vi "save_as.vi"(7 "calibration info":T1, 8 "Array":u16[][](array[numeric]), 9 "Camera":T2, 10 "Control Camera Properties 3":T3={"Packet Size"=1500, "Pixel Format"=17825797, "Gain in dB"=1.0, "Exposure Time in µs"=1500, "Stream Bytes per Second"=50000017} caption="Control Camera Properties" {"Stream Bytes per Second" min=1000000 max=124000000 step=100000 format="%.1p"; "Exposure Time in µs" min=21 max=153391689 format="%#.0f"; "Gain in dB" min=0.0 max=26.0 format="%#_2g"; "Pixel Format" items=["Mono 12 Packed"=17563654, "Mono 12"=17825797]}, 11 "path":path) -> (0 "saving error out":errorcluster, 2 "Name Time Date Out":string, 3 "Path out":path)   [LabVIEW 2014]
uses:
  type definitions/control camera properties.ctl
  type definitions/state machine enum.ctl
panel:
  out "Complete File Name Out":string
  in  "Time":bool
  in  "Date":bool
  in  "Name Time Date":string="im_spec" caption="Insert File Name"
  in  "Cancel Button":bool
  in  "Okay":bool
  in  "Path":path=path "C:/Users/loa/Documents/imaging-spectrometer/imaging-spectrometer/data"
  # "Tick box(es) to append time and/or date to file name:"
  # "Bytes"
  # "Trigger"
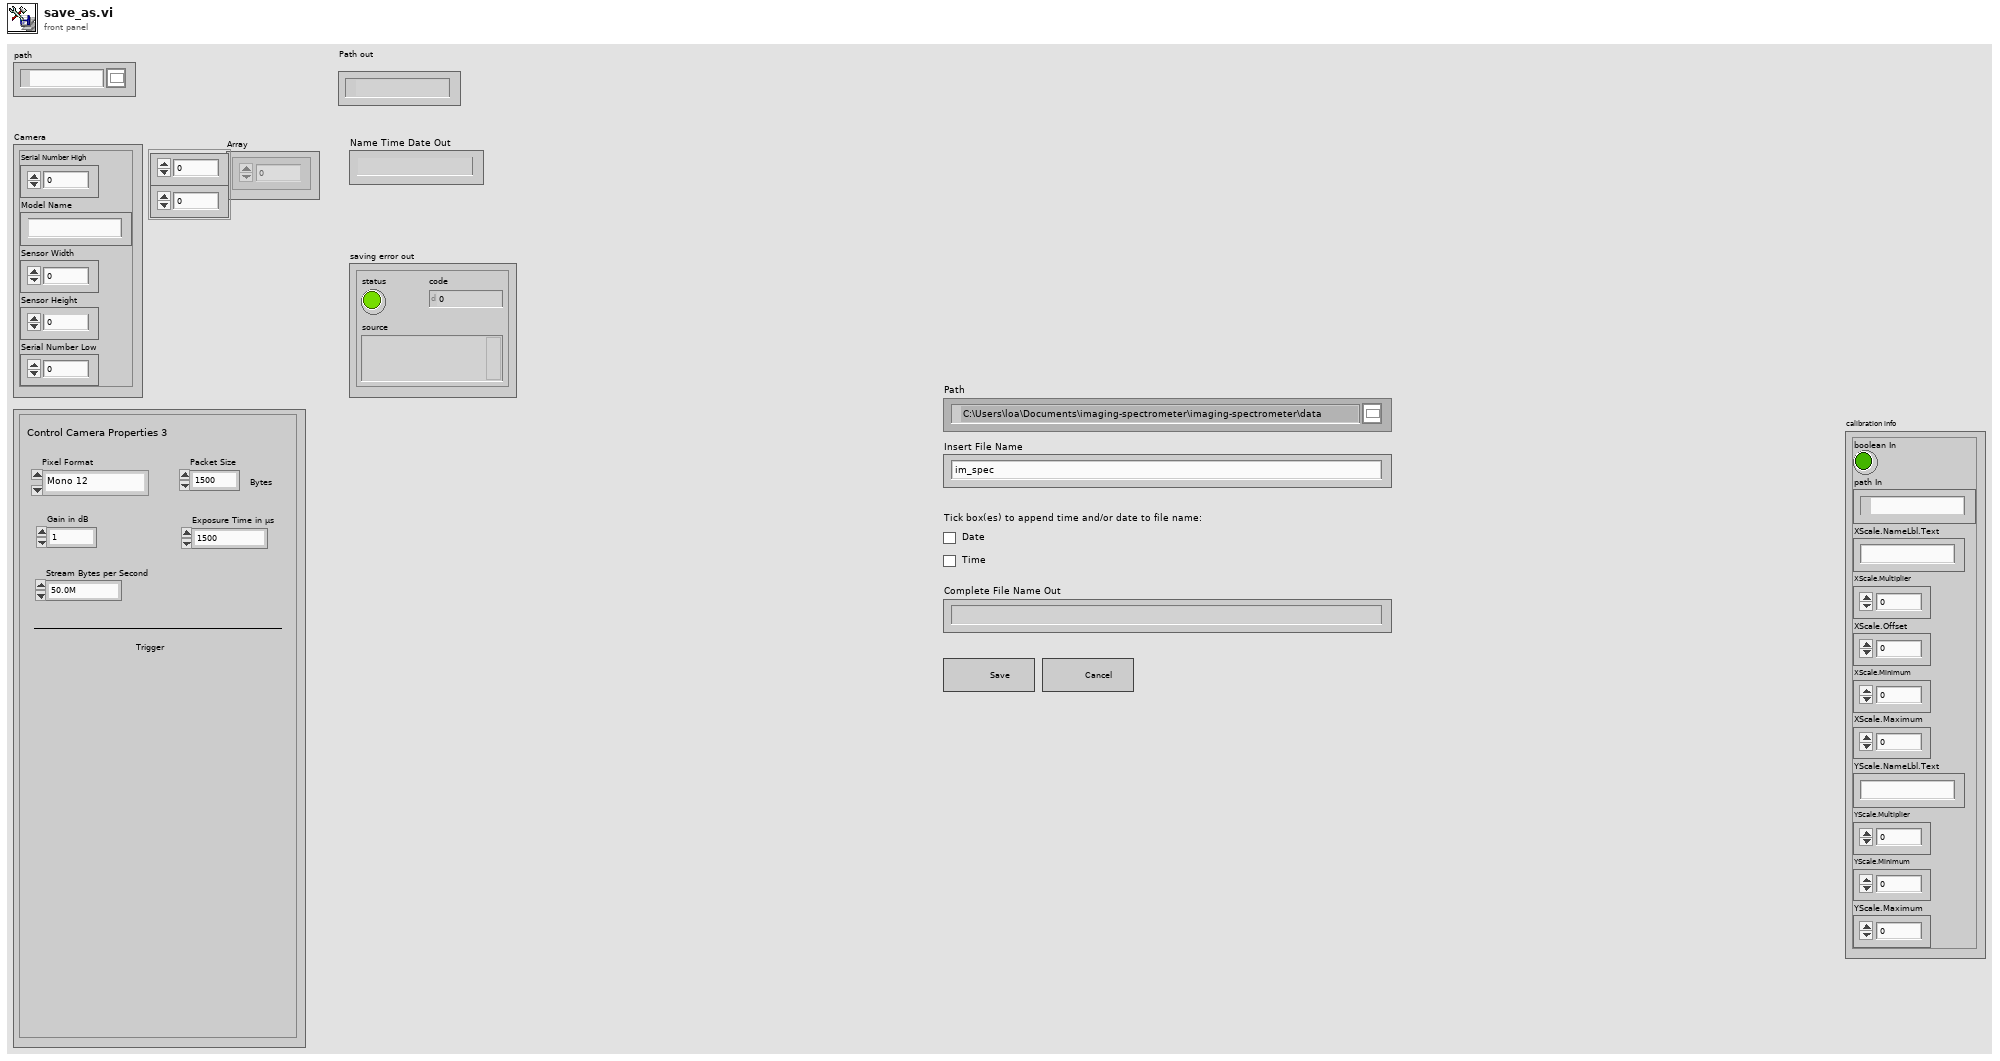
[diagram p1: front panel]
types:
  T1 = cluster{"boolean In":bool, "path In":path, "XScale.NameLbl.Text":string, "XScale.Multiplier":dbl, "XScale.Offset":dbl, "XScale.Minimum":dbl, "XScale.Maximum":dbl, "YScale.NameLbl.Text":string, "YScale.Multiplier":dbl, "YScale.Minimum":dbl, "YScale.Maximum":dbl}
  T2 = cluster{"Serial Number High":u32, "Model Name":string, "Sensor Width":u32, "Sensor Height":u32, "Serial Number Low":u32}
  T3 = typedef "control camera properties.ctl" = cluster{"Packet Size":u32, "Pixel Format":u32, "Gain in dB":dbl, "Exposure Time in µs":u32, "Stream Bytes per Second":u32}
  T4 = typedef "state machine enum.ctl" = enum16{"start", "select camera", "control camera properties", "calibration", "wait", "snap", "save", "save as", "grab", "error", "stop"}
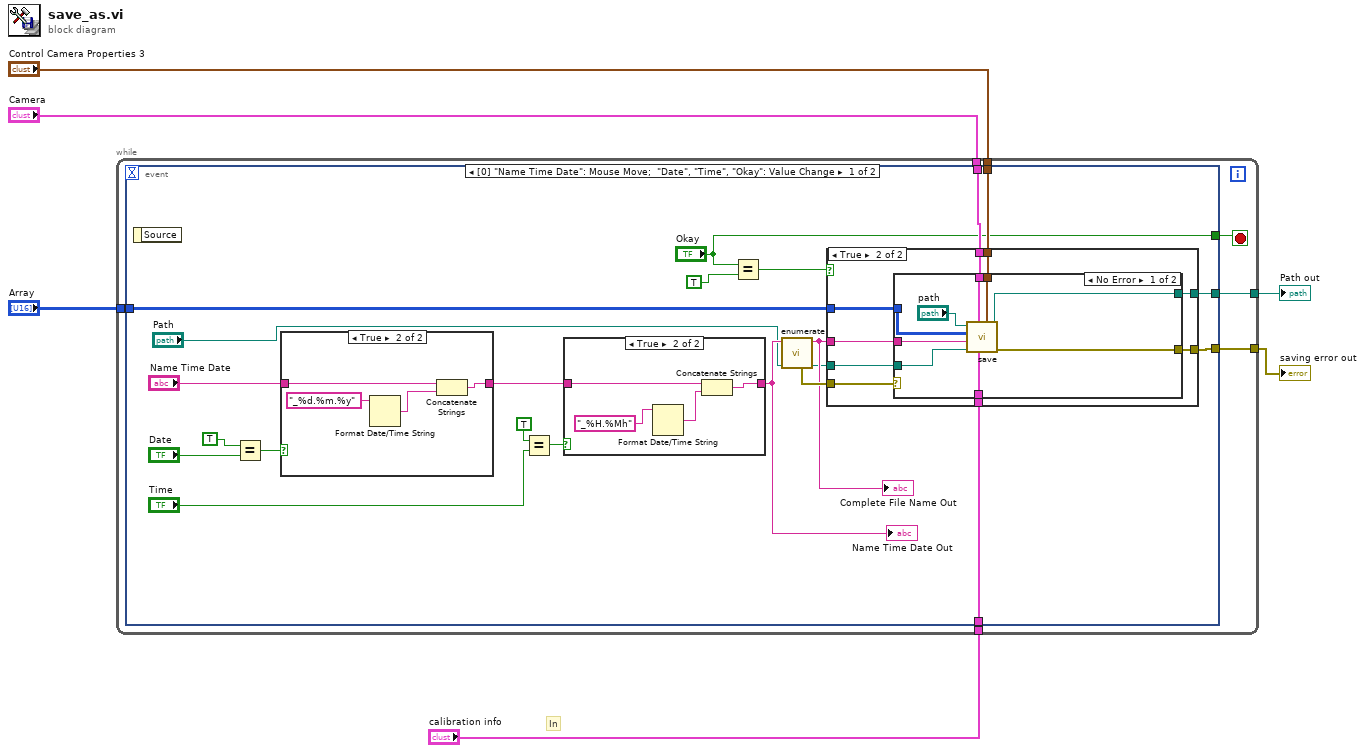
[diagram p0: block diagram]
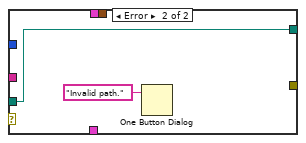
[diagram p3: hidden frame]
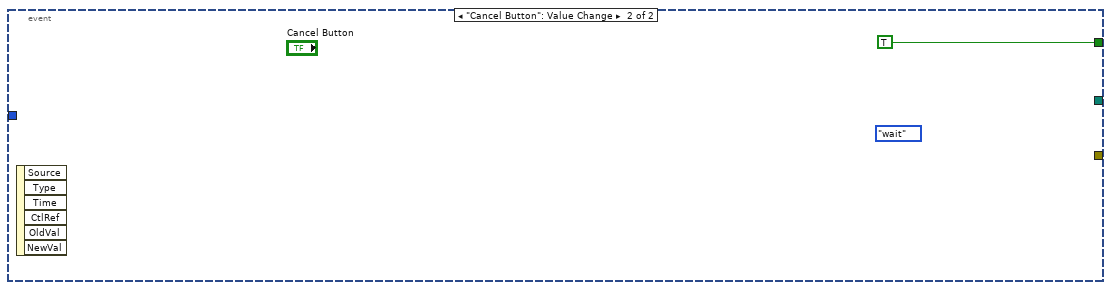
[diagram p6: hidden frame]
diagram:
  # "In"
  n1 = while {
    tunnel: "Control Camera Properties 3" -> [w12]
    tunnel: "Camera" -> [w11]
    tunnel: "Array" -> [w10]
    tunnel: [w9] -> w3
    tunnel: [w8] -> w2
    tunnel: "calibration info" -> [w7]
    stop <- w13 stop-if-true
    n2 = event shown="[0] \"Name Time Date\": Mouse Move;  \"Date\", \"Time\", \"Okay\": Value Change" {
      selector: _ -> [_ _]
      dyn-events: _ -> [_ _]
      timeout: _ -> [_ _]
      tunnel: ["Okay" TRUE] -> w13
      tunnel: w12 -> [w35 _]
      tunnel: w11 -> [w34 _]
      tunnel: w10 -> [w33 _]
      tunnel: [w32 _] -> w9
      tunnel: [w15 _] -> w8
      tunnel: w7 -> [w14 _]
      event "Name Time Date": Mouse Move; "Date", "Time", "Okay": Value Change {
        n3 = event-data() -> ()  [unwired: 1 in, 1 out]
        n4 = Equal?(x=TRUE, y="Date") -> (x = y?=w26:bool)
        n5 = case shown="True" w26 {
          tunnel: [w61 w64] -> w29
          tunnel: "Name Time Date" -> [w61 w62]
          frame False {
          }
          frame True {
            n6 = Format Date/Time String(time format string (%c)="_%d.%m.%y") -> (date/time string=w63:string)  [unwired: 2 in]
            n7 = Concatenate Strings(w62, w63) -> (w64:string)
          }
        }
        n8 = Equal?(x=TRUE, y="Time") -> (x = y?=w28:bool)
        n9 = case shown="True" w28 {
          tunnel: w29 -> [w56 w59]
          tunnel: [w56 w57] -> w21
          frame False {
          }
          frame True {
            n10 = Format Date/Time String(time format string (%c)="_%H.%Mh") -> (date/time string=w58:string)  [unwired: 2 in]
            n11 = Concatenate Strings(w59, w58) -> (w57:string)
          }
        }
        "Name Time Date Out" <- w21
        n12 = Equal?(x="Okay", y=TRUE) -> (x = y?=w17:bool)
        n13 = call "enumerate.vi"("Path In"="Path", "Name Time Date In"=w21) -> ("Path Out"=w18:path, "Complete File Name Out"=w19:string, "path error out"=w20:errorcluster)  [unwired: 7 in]
        "Complete File Name Out" <- w19
        n14 = case shown="True" w17 {
          tunnel: w35 -> [_ w44]
          tunnel: w34 -> [_ w43]
          tunnel: w33 -> [_ w42]
          tunnel: [_ w41] -> w32
          tunnel: w20 -> [_ w38]
          tunnel: w19 -> [_ w40]
          tunnel: w18 -> [_ w39]
          tunnel: [_ w37] -> w15
          tunnel: w14 -> [_ w36]
          frame False {
          }
          frame True {
            n15 = case shown="No Error" w38 {
              tunnel: w44 -> [w53 _]
              tunnel: w43 -> [w52 _]
              tunnel: w42 -> [w51 _]
              tunnel: [w50 w54] -> w41
              tunnel: w40 -> [w49 _]
              tunnel: w39 -> [w48 w54]
              tunnel: [w47 _] -> w37
              tunnel: w36 -> [w45 _]
              frame No Error {
                n16 = call "save.vi"("Control Camera Properties 3"=w53, "calibration info"=w45, "Camera"=w52, "Path"=w48, "Complete File Name In"=w49, "Array"=w51, "path"="path") -> ("saving error out"=w47:errorcluster, "Path out"=w50:path)  [unwired: 3 in]
              }
              frame Error {
                n17 = One Button Dialog(message="Invalid path.") -> ()  [unwired: 1 in, 1 out]
              }
            }
          }
        }
      }
      event "Cancel Button": Value Change {
        (unwired) state_machine_enum."wait" ("Zustände")
        n18 = event-data() -> ()  [unwired: 1 in, 6 out]
      }
    }
  }
  "Path out" <- w3
  "saving error out" <- w2
